vi "Front Panel.vi"(11 "GUI In":refnum<class "CRD Controls.lvclass">) -> ()   [LabVIEW 2015, in "CRD Controls.lvclass"]
uses:
  CRD Controls.lvclass
  Reusable/GUI/GUI.lvclass/GUI.ctl
  Reusable/Observer/Observer.lvclass/Observer.ctl
  CRDS/Data/cCRDS Data.lvclass
  Reusable/GUI/Accessors/Read RegEvent.vi
  Reusable/Observer/Read Data Queue.vi
  CRDS/Data/Read Humidifier T.vi
  CRDS/Data/Read Pressure.vi
  CRDS/Data/Read vData.vi
  CRDS/Data/Get Alicat Data.vi
  Reusable/Data/Data.lvclass
panel:
  in  "Med Humidity":T1
  in  "High Humidity":T1
  out "pidOut":cluster{"hum":sgl, "dry":sgl} caption="Humidifier PID \nOutput" {"dry" format="%#.2f"; "hum" format="%#.2f"}
  in  "orMFC":bool
  in  "lasEn":T2
  out "TRHin":cluster{"hum":sgl, "dry":sgl} caption="Humidifier \nTemperatures (degC)" {"dry" format="%#.2f"; "hum" format="%#.2f"}
  out "vaisalaData":T3 caption="Vaisala Data" {"ref 2"."TRH" format="%.2f"; "ref 2"."RH" format="%.2f"; "ref"."TRH" format="%.2f"; "ref"."RH" format="%.2f"; "dry"."TRH" format="%.2f"; "dry"."RH" format="%.2f"; "hum"."TRH" format="%.2g"; "hum"."RH" format="%.2g"}
  out "alctData":T4 caption="Alicat Data" {"purge"."P" format="%.2f"; "purge"."T" format="%.2f"; "purge"."Q" format="%.2f"; "hRH"."P" format="%.2f"; "hRH"."T" format="%.2f"; "hRH"."Q" format="%.2f"; "mRH"."P" format="%.2f"; "mRH"."T" format="%.2f"; "mRH"."Q" format="%.2f"; "dry"."P" format="%.2f"; "dry"."T" format="%.2f"; "dry"."Q" format="%.2f"; "denude"."P" format="%.2f"; "denude"."T" format="%.2f"; "denude"."Q" format="%.2f"}
  out "P":T5 caption="Pressure (mb)" {"ref 2" format="%#.2f"; "ref" format="%#.2f"; "dry" format="%#.2f"; "hum" format="%#.2f"}
  in  "Laser Controls":cluster{"f (Hz)":dbl, "Duty Cycle (%)":dbl}
  in  "crdFlows":T6 caption="Flow Rate Setpoints (LPM)" {"purge" max=5 format="%.2f"; "hRH" max=5 format="%.2f"; "mRH" max=5 format="%.2f"; "dry" max=5 format="%.2f"; "denude" max=5 format="%.2f"}
  # "CRD Controls"
  # "CRD Controller Data"
  # "Laser Enable"
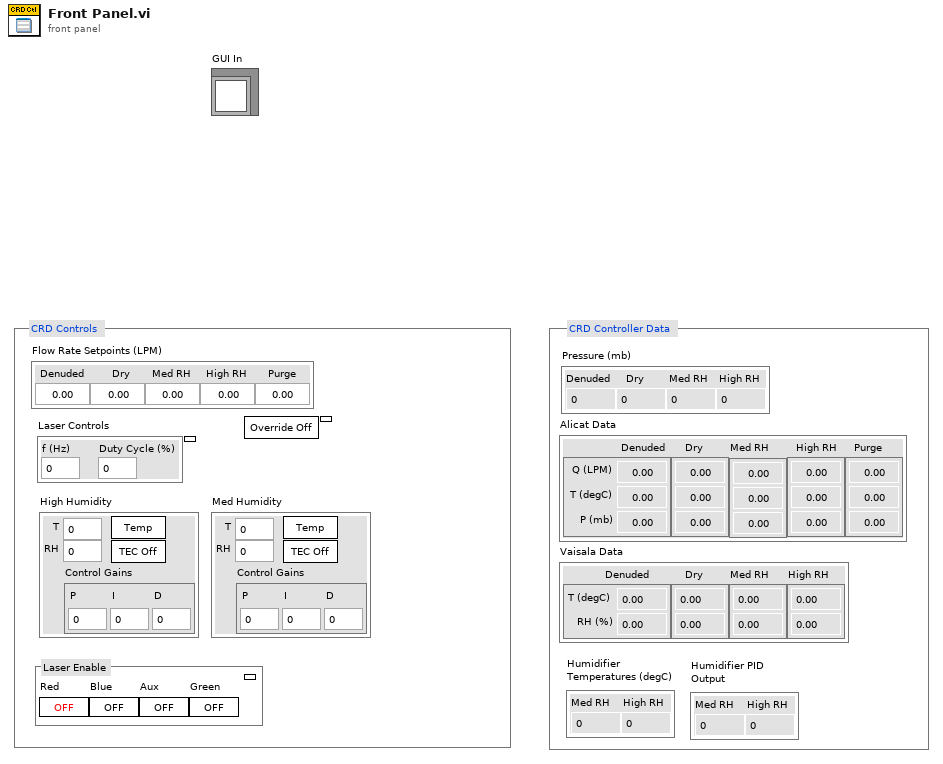
[diagram p1: front panel]
types:
  T1 = cluster{"T":dbl, "RH":dbl, "enable":bool, "ctl":bool, "Ctl Gains":cluster{"P":sgl, "I":sgl, "D":sgl}}
  T2 = cluster{"red":bool, "Blue":bool, "Aux":bool, "Green":bool}
  T3 = cluster{"hum":cluster{"RH":sgl, "TRH":sgl}, "dry":cluster{"RH":sgl, "TRH":sgl}, "ref":cluster{"RH":sgl, "TRH":sgl}, "ref 2":cluster{"RH":sgl, "TRH":sgl}}
  T4 = cluster{"denude":cluster{"Q":sgl, "T":sgl, "P":sgl}, "dry":cluster{"Q":sgl, "T":sgl, "P":sgl}, "mRH":cluster{"Q":sgl, "T":sgl, "P":sgl}, "hRH":cluster{"Q":sgl, "T":sgl, "P":sgl}, "purge":cluster{"Q":sgl, "T":sgl, "P":sgl}}
  T5 = cluster{"hum":sgl, "dry":sgl, "ref":sgl, "ref 2":sgl}
  T6 = cluster{"denude":sgl, "dry":sgl, "mRH":sgl, "hRH":sgl, "purge":sgl}
  T7 = enum8{"Enabled", "Disabled", "Disabled and Grayed Out"}
  T8 = cluster{"Array of Single[0]":sgl, "Array of Single[1]":sgl, "Array of Single[2]":sgl}
  T9 = cluster{"Numeric":sgl, "Numeric":sgl, "Numeric":sgl, "Numeric":sgl, "Numeric":sgl}
  T10 = cluster{"P":sgl, "T":sgl, "Q":sgl, "Q0":sgl, "Qsp":sgl}[]
  T11 = cluster{"Pressure[0]":sgl, "Pressure[1]":sgl, "Pressure[2]":sgl, "Pressure[3]":sgl}
  T12 = cluster{"vData[0]":cluster{"TRH":dbl, "RH":dbl}, "vData[1]":cluster{"TRH":dbl, "RH":dbl}, "vData[2]":cluster{"TRH":dbl, "RH":dbl}, "vData[3]":cluster{"TRH":dbl, "RH":dbl}}
  T13 = cluster{"P":sgl, "T":sgl, "Q":sgl, "Q0":sgl, "Qsp":sgl}
  T14 = cluster{"[0]":cluster{"Q":sgl, "T":sgl, "P":sgl}, "[1]":cluster{"Q":sgl, "T":sgl, "P":sgl}, "[2]":cluster{"Q":sgl, "T":sgl, "P":sgl}, "[3]":cluster{"Q":sgl, "T":sgl, "P":sgl}, "[4]":cluster{"Q":sgl, "T":sgl, "P":sgl}}
  T15 = cluster{"Array of Single[0]":sgl, "Array of Single[1]":sgl}
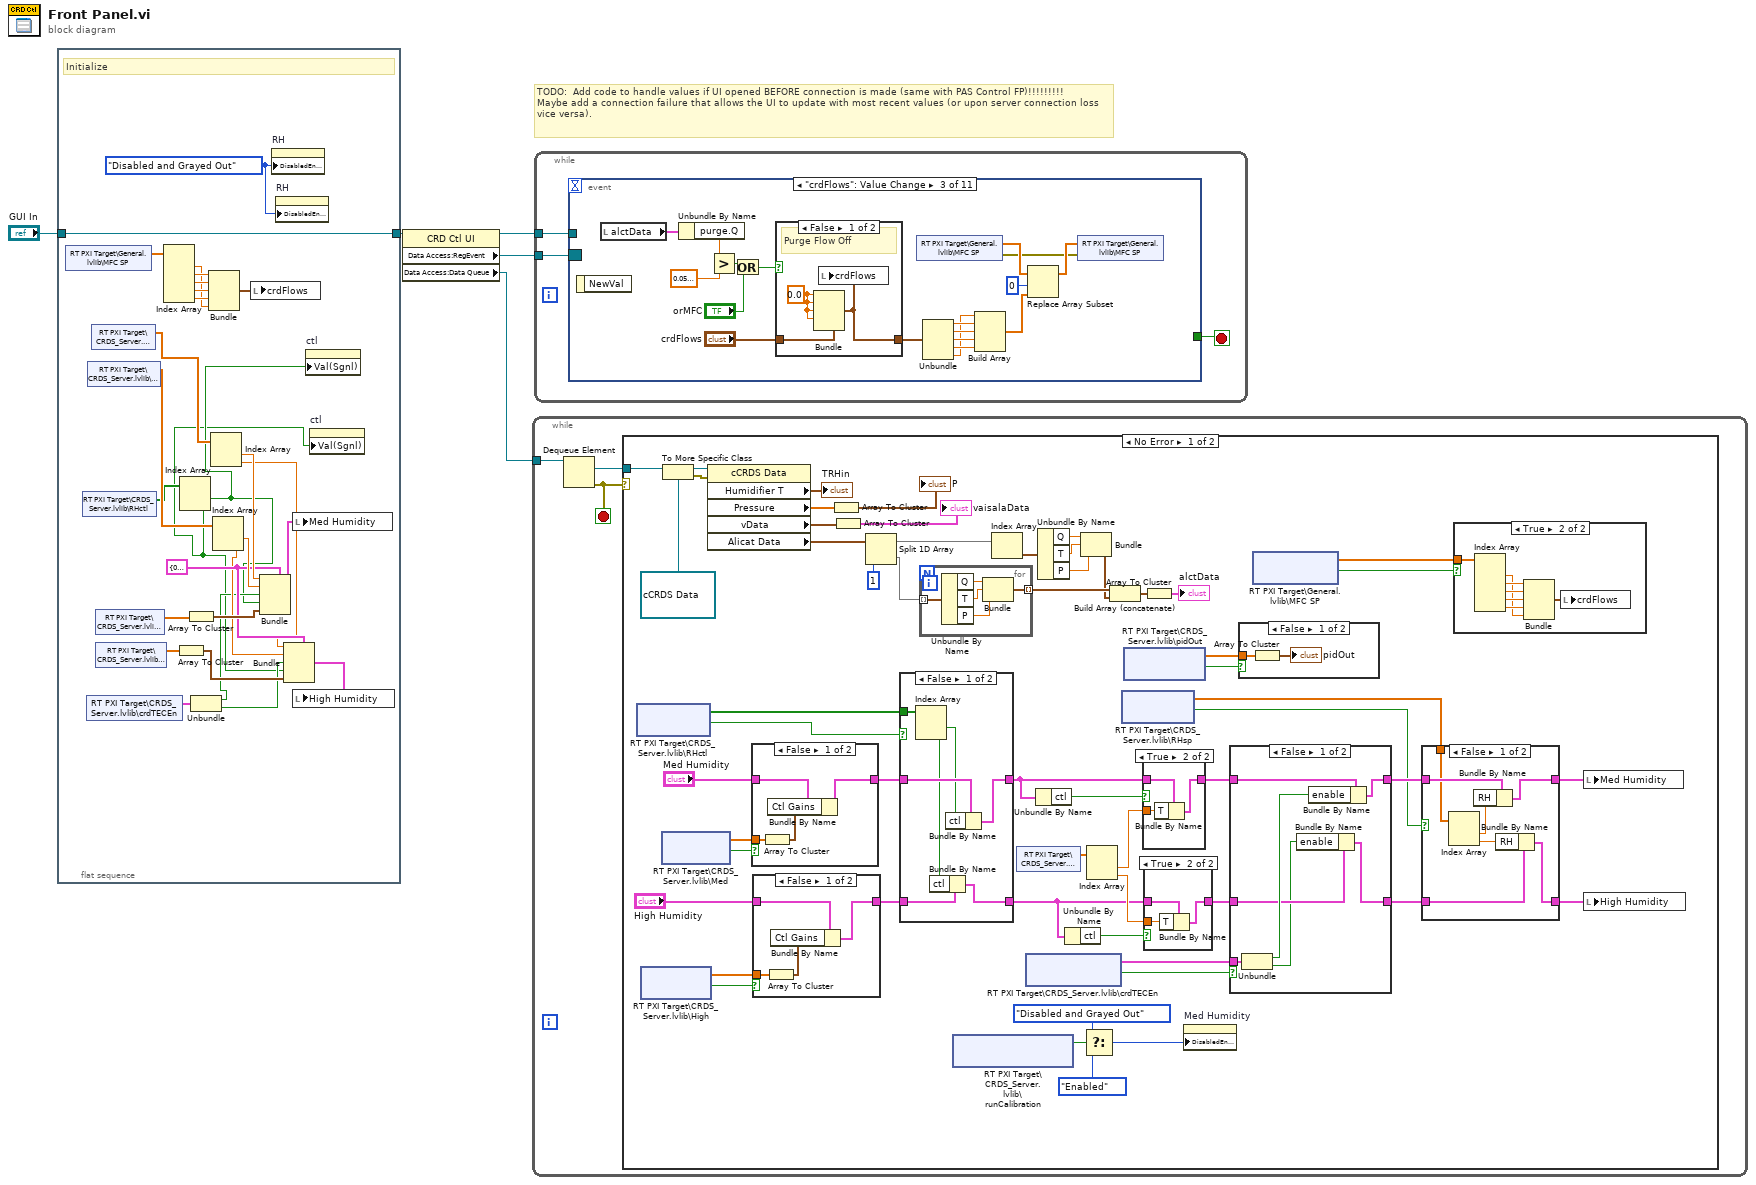
[diagram p0: block diagram]
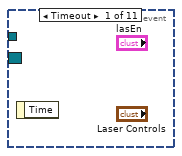
[diagram p2: hidden frame]
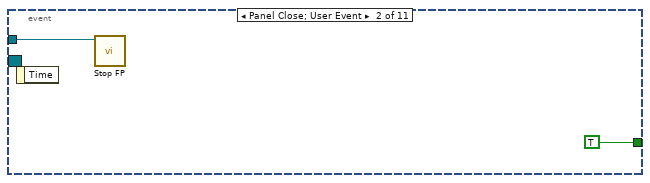
[diagram p3: hidden frame]
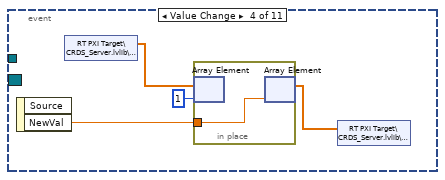
[diagram p5: hidden frame]
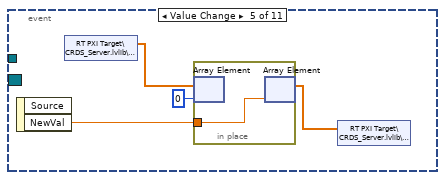
[diagram p6: hidden frame]
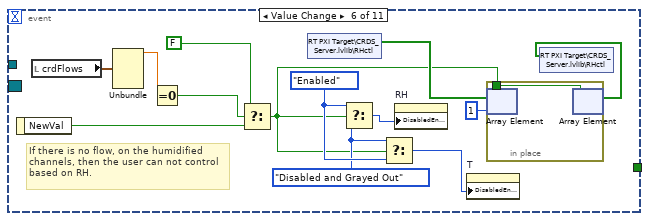
[diagram p7: hidden frame]
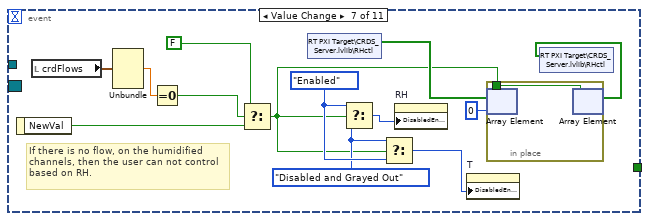
[diagram p8: hidden frame]
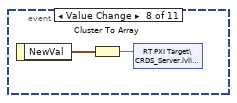
[diagram p9: hidden frame]
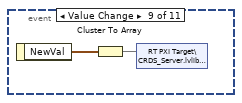
[diagram p10: hidden frame]
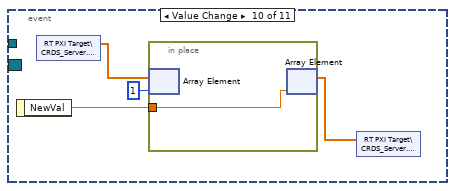
[diagram p11: hidden frame]
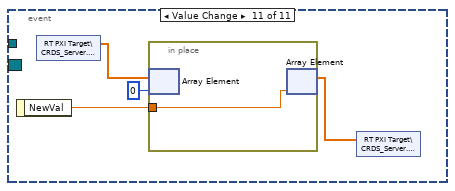
[diagram p12: hidden frame]
diagram:
  # "TODO:  Add code to handle values if UI opened BEFORE connection is made (same with PAS Control FP)!!!!!!!!!\nMaybe add a connection failure that allows the UI to update with most recent values (or upon server connection loss vice versa)."
  n1 = flat-sequence {
    tunnel: "GUI In" -> [w26]
    tunnel: [w26] -> w4
    frame #0 {
      w8 = T7."Disabled and Grayed Out" ("Disabled")
      w18 = T1 {"T"=0.0, "RH"=0.0, "enable"=FALSE, "ctl"=FALSE, "Ctl Gains"={"P"=3.0, "I"=10.0, "D"=0.1}} ("High Humidity")
      # "Initialize"
      n2 = shared-variable "RT PXI Target\\General.lvlib\\MFC SP"() -> (w33:sgl[])  [unwired: 1 in, 1 out]
      n3 = shared-variable "RT PXI Target\\CRDS_Server.lvlib\\RHctl"() -> (w14:bool[])  [unwired: 1 in, 1 out]
      n4 = shared-variable "RT PXI Target\\CRDS_Server.lvlib\\crdTECEn"() -> (w13:cluster{"med":bool, "high":bool})  [unwired: 1 in, 1 out]
      n5 = shared-variable "RT PXI Target\\CRDS_Server.lvlib\\RHsp"() -> (w22:sgl[])  [unwired: 1 in, 1 out]
      n6 = shared-variable "RT PXI Target\\CRDS_Server.lvlib\\Tsp"() -> (w23:sgl[])  [unwired: 1 in, 1 out]
      n7 = shared-variable "RT PXI Target\\CRDS_Server.lvlib\\Med"() -> (w25:sgl[])  [unwired: 1 in, 1 out]
      n8 = shared-variable "RT PXI Target\\CRDS_Server.lvlib\\High"() -> (w24:sgl[])  [unwired: 1 in, 1 out]
      n9 = Index Array(array=w33) -> (element #1=w28:sgl, element #2=w32:sgl, element #3=w31:sgl, element #4=w30:sgl, element #5=w29:sgl)  [unwired: 5 in]
      n10 = Array To Cluster(array=w24) -> (cluster=w17:T8)
      n11 = Index Array(array=w14) -> (element #1=w7:bool, element #2=w6:bool)  [unwired: 2 in]
      n12 = Array To Cluster(array=w25) -> (cluster=w21:T8)
      n13 = Unbundle(w13) -> ("med"=w12:bool, "high"=w11:bool)
      n14 = Bundle("Numeric"=w32, "Numeric"=w31, "Numeric"=w30, "Numeric"=w29, "Numeric"=w28) -> (w27:T9)  [unwired: 1 in]
      n15 = Index Array(array=w23) -> (element #1=w20:sgl, element #2=w16:sgl)  [unwired: 2 in]
      n16 = Index Array(array=w22) -> (element #1=w19:sgl, element #2=w15:sgl)  [unwired: 2 in]
      n17 = local write "crdFlows"(w27) -> ()
      n18 = Bundle(cluster=w18, "T"=w20, "RH"=w19, "enable"=w12, "ctl"=w7, "Ctl Gains"=w21) -> (w9:T1)
      n19 = property on="RH" class="DigNum (strict)"("DisabledEnum"=w8) -> ()  [unwired: 2 in, 2 out]
      n20 = property on="RH" class="DigNum (strict)"("DisabledEnum"=w8) -> ()  [unwired: 2 in, 2 out]
      n21 = Bundle(cluster=w18, "T"=w16, "RH"=w15, "enable"=w11, "ctl"=w6, "Ctl Gains"=w17) -> (w10:T1)
      n22 = local write "Med Humidity"(w9) -> ()
      n23 = local write "High Humidity"(w10) -> ()
      n24 = property on="ctl" class="Bool (strict)"("Val(Sgnl)"=w7) -> ()  [unwired: 2 in, 2 out]
      n25 = property on="ctl" class="Bool (strict)"("Val(Sgnl)"=w6) -> ()  [unwired: 2 in, 2 out]
    }
  }
  n26 = property class="CRD Ctl UI"(reference=w4) -> (reference out=w1:refnum<class "CRD Controls.lvclass">, "Data Access:RegEvent"=w3:refnum<event-registration>, "Data Access:Data Queue"=w2:refnum<queue>)  [unwired: 1 in, 1 out]
  n27 = while {
    tunnel: w2 -> [w36]
    stop <- w35 stop-if-true
    n28 = Dequeue Element(queue=w36) -> (element=w34:refnum<data-value>, error out=w35:errorcluster)  [unwired: 2 in, 2 out]
    n29 = case shown="No Error" w35 {
      tunnel: w34 -> [w75 _]
      frame No Error {
        n30 = shared-variable "RT PXI Target\\CRDS_Server.lvlib\\RHctl"() -> (w62:bool[], w64:bool)  [unwired: 2 in, 1 out]
        n31 = shared-variable "RT PXI Target\\CRDS_Server.lvlib\\High"() -> (w70:sgl[], w71:bool)  [unwired: 2 in, 1 out]
        n32 = shared-variable "RT PXI Target\\CRDS_Server.lvlib\\Med"() -> (w69:sgl[], w68:bool)  [unwired: 2 in, 1 out]
        n33 = To More Specific Class(target class=refnum<data-value> refnum ("element"), reference=w75) -> (specific class reference=w74:refnum<data-value>, error out=w73:errorcluster)  [unwired: 1 in]
        n34 = property class="cCRDS Data"(reference=w74, error in=w73) -> ("Humidifier T"=→"TRHin":cluster{"Hum 1":sgl, "Hum 2":sgl}, "Pressure"=w86:sgl[], "vData"=w85:cluster{"TRH":dbl, "RH":dbl}[], "Alicat Data"=w81:T10)  [unwired: 2 out]
        n35 = case shown="False" w68 {
          tunnel: w69 -> [w140 _]
          tunnel: "Med Humidity" -> [w139 w141]
          tunnel: [w137 w141] -> w60
          frame False {
            n36 = Array To Cluster(array=w140) -> (cluster=w138:T8)
            n37 = Bundle By Name(cluster=w139, "Ctl Gains"=w138) -> (w137:T1)
          }
          frame True {
          }
        }
        n38 = case shown="False" w71 {
          tunnel: w70 -> [w145 _]
          tunnel: "High Humidity" -> [w144 w146]
          tunnel: [w142 w146] -> w63
          frame False {
            n39 = Array To Cluster(array=w145) -> (cluster=w143:T8)
            n40 = Bundle By Name(cluster=w144, "Ctl Gains"=w143) -> (w142:T1)
          }
          frame True {
          }
        }
        n41 = Array To Cluster(array=w86) -> (cluster=→"P":T11)
        n42 = Array To Cluster(array=w85) -> (cluster=→"vaisalaData":T12)
        n43 = Split 1D Array(array=w81, index=1) -> (first subarray=w91:T10, second subarray=w92:T10)
        n44 = case shown="False" w64 {
          tunnel: w63 -> [w132 w134]
          tunnel: [w131 w134] -> w54
          tunnel: w62 -> [w129 _]
          tunnel: w60 -> [w130 w133]
          tunnel: [w126 w133] -> w53
          frame False {
            n45 = Index Array(array=w129) -> (element #1=w127:bool, element #2=w128:bool)  [unwired: 2 in]
            n46 = Bundle By Name(cluster=w132, "ctl"=w128) -> (w131:T1)
            n47 = Bundle By Name(cluster=w130, "ctl"=w127) -> (w126:T1)
          }
          frame True {
          }
        }
        n48 = for {
          tunnel: w92 -> [w151] mode=indexing
          tunnel: [w150] -> w90 mode=indexing
          n49 = Unbundle By Name(w151) -> ("Q"=w149:sgl, "T"=w148:sgl, "P"=w147:sgl)
          n50 = Bundle("Q"=w149, "T"=w148, "P"=w147) -> (w150:cluster{"Q":sgl, "T":sgl, "P":sgl})  [unwired: 1 in]
        }
        n51 = shared-variable "RT PXI Target\\CRDS_Server.lvlib\\runCalibration"() -> (w42:bool)  [unwired: 2 in, 2 out]
        n52 = Index Array(array=w91) -> (element=w87:T13)  [unwired: 1 in]
        n53 = shared-variable "RT PXI Target\\CRDS_Server.lvlib\\Tsp"() -> (w57:sgl[])  [unwired: 1 in, 1 out]
        n54 = shared-variable "RT PXI Target\\CRDS_Server.lvlib\\crdTECEn"() -> (w49:cluster{"med":bool, "high":bool}, w52:bool)  [unwired: 2 in, 1 out]
        n55 = Unbundle By Name(w53) -> ("ctl"=w59:bool)
        n56 = Unbundle By Name(w87) -> ("Q"=w84:sgl, "T"=w83:sgl, "P"=w82:sgl)
        n57 = Unbundle By Name(w54) -> ("ctl"=w58:bool)
        n58 = Bundle("Q"=w84, "T"=w83, "P"=w82) -> (w80:cluster{"Q":sgl, "T":sgl, "P":sgl})  [unwired: 1 in]
        n59 = Select(t=T7."Disabled and Grayed Out" ("Disabled"), s=w42, f=T7."Enabled" ("Disabled")) -> (s? t:f=w39:T7)
        n60 = Index Array(array=w57) -> (element #1=w56:sgl, element #2=w55:sgl)  [unwired: 2 in]
        n61 = Build Array (concatenate)(w90, w80) -> (w89:cluster{"Q":sgl, "T":sgl, "P":sgl}[])
        n62 = shared-variable "RT PXI Target\\CRDS_Server.lvlib\\RHsp"() -> (w45:sgl[], w46:bool)  [unwired: 2 in, 1 out]
        n63 = shared-variable "RT PXI Target\\CRDS_Server.lvlib\\pidOut"() -> (w67:sgl[], w66:bool)  [unwired: 2 in, 1 out]
        n64 = case shown="True" w59 {
          tunnel: w56 -> [_ w124]
          tunnel: w53 -> [w122 w125]
          tunnel: [w122 w123] -> w51
          frame False {
          }
          frame True {
            n65 = Bundle By Name(cluster=w125, "T"=w124) -> (w123:T1)
          }
        }
        n66 = Array To Cluster(array=w89) -> (cluster=→"alctData":T14)
        n67 = case shown="True" w58 {
          tunnel: w55 -> [_ w120]
          tunnel: w54 -> [w118 w121]
          tunnel: [w118 w119] -> w50
          frame False {
          }
          frame True {
            n68 = Bundle By Name(cluster=w121, "T"=w120) -> (w119:T1)
          }
        }
        n69 = property on="Med Humidity" class="Clust (strict)"("DisabledEnum"=w39) -> ()  [unwired: 2 in, 2 out]
        n70 = case shown="False" w52 {
          tunnel: w51 -> [w114 w117]
          tunnel: w50 -> [w111 w116]
          tunnel: [w113 w117] -> w48
          tunnel: [w109 w116] -> w47
          tunnel: w49 -> [w115 _]
          frame False {
            n71 = Unbundle(w115) -> ("med"=w112:bool, "high"=w110:bool)
            n72 = Bundle By Name(cluster=w111, "enable"=w110) -> (w109:T1)
            n73 = Bundle By Name(cluster=w114, "enable"=w112) -> (w113:T1)
          }
          frame True {
          }
        }
        n74 = case shown="False" w66 {
          tunnel: w67 -> [w136 _]
          frame False {
            n75 = Array To Cluster(array=w136) -> (cluster=→"pidOut":T15)
          }
          frame True {
          }
        }
        n76 = shared-variable "RT PXI Target\\General.lvlib\\MFC SP"() -> (w37:sgl[], w38:bool)  [unwired: 2 in, 1 out]
        n77 = case shown="False" w46 {
          tunnel: w48 -> [w106 w108]
          tunnel: [w105 w108] -> w43
          tunnel: [w104 w107] -> w44
          tunnel: w47 -> [w103 w107]
          tunnel: w45 -> [w102 _]
          frame False {
            n78 = Index Array(array=w102) -> (element #1=w101:sgl, element #2=w100:sgl)  [unwired: 2 in]
            n79 = Bundle By Name(cluster=w106, "RH"=w101) -> (w105:T1)
            n80 = Bundle By Name(cluster=w103, "RH"=w100) -> (w104:T1)
          }
          frame True {
          }
        }
        n81 = case shown="True" w38 {
          tunnel: w37 -> [_ w99]
          frame False {
          }
          frame True {
            n82 = Index Array(array=w99) -> (element #1=w94:sgl, element #2=w98:sgl, element #3=w97:sgl, element #4=w96:sgl, element #5=w95:sgl)  [unwired: 5 in]
            n83 = Bundle("Numeric"=w98, "Numeric"=w97, "Numeric"=w96, "Numeric"=w95, "Numeric"=w94) -> (w93:T9)  [unwired: 1 in]
            n84 = local write "crdFlows"(w93) -> ()
          }
        }
        n85 = local write "Med Humidity"(w43) -> ()
        n86 = local write "High Humidity"(w44) -> ()
      }
      frame Error {
      }
    }
  }
  n87 = while {
    tunnel: w3 -> [w153]
    tunnel: w1 -> [w152]
    stop <- w154 stop-if-true
    n88 = event shown="[2] \"crdFlows\": Value Change" {
      selector: w153 -> [_ _ _ _ _ _ _ _ _ _ _]
      dyn-events: _ -> [_ _ _ _ _ _ _ _ _ _ _]
      timeout: _ -> [_ _ _ _ _ _ _ _ _ _ _]
      tunnel: [_ TRUE _ _ _ _ _ _ _ _ _] -> w154
      tunnel: w152 -> [_ w155 _ _ _ _ _ _ _ _ _]
      event Timeout {
        n89 = event-data() -> ()  [unwired: 1 in, 1 out]
      }
      event Panel Close; User Event {
        n90 = event-data() -> ()  [unwired: 1 in, 1 out]
        n91 = call-dynamic "Stop FP.vi"("GUI in"=w155) -> ()  [unwired: 9 in, 2 out]
      }
      event "crdFlows": Value Change {
        n92 = event-data() -> ()  [unwired: 1 in, 1 out]
        n93 = local read "alctData"() -> (w161:T4)
        n94 = Unbundle By Name(w161) -> ("purge.Q"=w163:sgl)
        n95 = Greater?(x=w163, y=sgl 0.05) -> (0:w158:bool)
        n96 = Or(x=w158, y="orMFC") -> (x .or. y?=w157:bool)
        n97 = case shown="False" w157 {
          tunnel: "crdFlows" -> [w177 w178]
          tunnel: [w175 w178] -> w162
          frame False {
            w176 = sgl 0.0 ("denude")
            # "Purge Flow Off"
            n98 = Bundle(cluster=w177, "denude"=w176, "dry"=w176, "mRH"=w176, "hRH"=w176) -> (w175:T6)  [unwired: 1 in]
            n99 = local write "crdFlows"(w175) -> ()
          }
          frame True {
          }
        }
        n100 = shared-variable "RT PXI Target\\General.lvlib\\MFC SP"() -> (w171:sgl[], error out=w165:errorcluster)  [unwired: 1 in]
        n101 = Unbundle(w162) -> ("denude"=w167:sgl, "dry"=w168:sgl, "mRH"=w169:sgl, "hRH"=w170:sgl, "purge"=w166:sgl)
        n102 = Build Array(w166, w167, w168, w169, w170) -> (w173:sgl[])
        n103 = Replace Array Subset(array=w171, new element=w173, index=0) -> (w172:sgl[])
        n104 = shared-variable "RT PXI Target\\General.lvlib\\MFC SP"(w172, error in=w165) -> ()  [unwired: 1 out]
      }
      event "High Humidity.RH": Value Change {
        n105 = event-data() -> ("NewVal"=w179:dbl)  [unwired: 1 in, 1 out]
        n106 = shared-variable "RT PXI Target\\CRDS_Server.lvlib\\RHsp"() -> (w182:sgl[])  [unwired: 1 in, 1 out]
        n107 = in-place {
          in-place-border: w179 -> [w183]
          n108 = in-place-array #1(w182, 1) -> ()  [unwired: 1 out]
          n109 = in-place-array #1(w183) -> (w181:sgl[])  [unwired: 1 out]
        }
        n110 = shared-variable "RT PXI Target\\CRDS_Server.lvlib\\RHsp"(w181) -> ()  [unwired: 1 in, 1 out]
      }
      event "Med Humidity.RH": Value Change {
        n111 = event-data() -> ("NewVal"=w184:dbl)  [unwired: 1 in, 1 out]
        n112 = shared-variable "RT PXI Target\\CRDS_Server.lvlib\\RHsp"() -> (w187:sgl[])  [unwired: 1 in, 1 out]
        n113 = in-place {
          in-place-border: w184 -> [w188]
          n114 = in-place-array #2(w187, 0) -> ()  [unwired: 1 out]
          n115 = in-place-array #2(w188) -> (w186:sgl[])  [unwired: 1 out]
        }
        n116 = shared-variable "RT PXI Target\\CRDS_Server.lvlib\\RHsp"(w186) -> ()  [unwired: 1 in, 1 out]
      }
      event "High Humidity.ctl": Value Change {
        w199 = T7."Disabled and Grayed Out" ("Disabled")
        w200 = T7."Enabled" ("Disabled")
        # "If there is no flow, on the humidified channels, then the user can not control based on RH."
        n117 = event-data() -> ("NewVal"=w196:bool)  [unwired: 1 in]
        n118 = local read "crdFlows"() -> (w197:T6)
        n119 = Unbundle(w197) -> ("denude"=w189:sgl)  [unwired: 4 out]
        n120 = Equal To 0?(x=w189) -> (x = 0?=w198:bool)
        n121 = Select(t=FALSE, s=w198, f=w196) -> (s? t:f=w192:bool)
        n122 = shared-variable "RT PXI Target\\CRDS_Server.lvlib\\RHctl"() -> (w195:bool[])  [unwired: 1 in, 1 out]
        n123 = Select(t=w200, s=w192, f=w199) -> (s? t:f=w191:T7)
        n124 = Select(t=w199, s=w192, f=w200) -> (s? t:f=w190:T7)
        n125 = property on="RH" class="DigNum (strict)"("DisabledEnum"=w191) -> ()  [unwired: 2 in, 2 out]
        n126 = property on="T" class="DigNum (strict)"("DisabledEnum"=w190) -> ()  [unwired: 2 in, 2 out]
        n127 = in-place {
          in-place-border: w192 -> [w202]
          n128 = in-place-array #3(w195, 1) -> ()  [unwired: 1 out]
          n129 = in-place-array #3(w202) -> (w193:bool[])  [unwired: 1 out]
        }
        n130 = shared-variable "RT PXI Target\\CRDS_Server.lvlib\\RHctl"(w193) -> ()  [unwired: 1 in, 1 out]
      }
      event "Med Humidity.ctl": Value Change {
        w213 = T7."Disabled and Grayed Out" ("Disabled")
        w214 = T7."Enabled" ("Disabled")
        # "If there is no flow, on the humidified channels, then the user can not control based on RH."
        n131 = event-data() -> ("NewVal"=w210:bool)  [unwired: 1 in]
        n132 = local read "crdFlows"() -> (w211:T6)
        n133 = Unbundle(w211) -> ("mRH"=w203:sgl)  [unwired: 4 out]
        n134 = Equal To 0?(x=w203) -> (x = 0?=w212:bool)
        n135 = Select(t=FALSE, s=w212, f=w210) -> (s? t:f=w206:bool)
        n136 = shared-variable "RT PXI Target\\CRDS_Server.lvlib\\RHctl"() -> (w209:bool[])  [unwired: 1 in, 1 out]
        n137 = Select(t=w214, s=w206, f=w213) -> (s? t:f=w205:T7)
        n138 = Select(t=w213, s=w206, f=w214) -> (s? t:f=w204:T7)
        n139 = property on="RH" class="Digital (strict)"("DisabledEnum"=w205) -> ()  [unwired: 2 in, 2 out]
        n140 = property on="T" class="Digital (strict)"("DisabledEnum"=w204) -> ()  [unwired: 2 in, 2 out]
        n141 = in-place {
          in-place-border: w206 -> [w216]
          n142 = in-place-array #4(w209, 0) -> ()  [unwired: 1 out]
          n143 = in-place-array #4(w216) -> (w207:bool[])  [unwired: 1 out]
        }
        n144 = shared-variable "RT PXI Target\\CRDS_Server.lvlib\\RHctl"(w207) -> ()  [unwired: 1 in, 1 out]
      }
      event "Med Humidity.Ctl Gains": Value Change {
        n145 = event-data() -> ("NewVal"=w218:cluster{"P":sgl, "I":sgl, "D":sgl})  [unwired: 1 in]
        n146 = Cluster To Array(cluster=w218) -> (array=w217:sgl[])
        n147 = shared-variable "RT PXI Target\\CRDS_Server.lvlib\\Med"(w217) -> ()  [unwired: 1 in, 1 out]
      }
      event "High Humidity.Ctl Gains": Value Change {
        n148 = event-data() -> ("NewVal"=w219:cluster{"P":sgl, "I":sgl, "D":sgl})  [unwired: 1 in]
        n149 = Cluster To Array(cluster=w219) -> (array=w220:sgl[])
        n150 = shared-variable "RT PXI Target\\CRDS_Server.lvlib\\High"(w220) -> ()  [unwired: 1 in, 1 out]
      }
      event "High Humidity.T": Value Change {
        n151 = event-data() -> ("NewVal"=w222:dbl)  [unwired: 1 in]
        n152 = shared-variable "RT PXI Target\\CRDS_Server.lvlib\\Tsp"() -> (w224:sgl[])  [unwired: 1 in, 1 out]
        n153 = in-place {
          in-place-border: w222 -> [w225]
          n154 = in-place-array #5(w224, 1) -> ()  [unwired: 1 out]
          n155 = in-place-array #5(w225) -> (w221:sgl[])  [unwired: 1 out]
        }
        n156 = shared-variable "RT PXI Target\\CRDS_Server.lvlib\\Tsp"(w221) -> ()  [unwired: 1 in, 1 out]
      }
      event "Med Humidity.T": Value Change {
        n157 = event-data() -> ("NewVal"=w227:dbl)  [unwired: 1 in]
        n158 = shared-variable "RT PXI Target\\CRDS_Server.lvlib\\Tsp"() -> (w229:sgl[])  [unwired: 1 in, 1 out]
        n159 = in-place {
          in-place-border: w227 -> [w230]
          n160 = in-place-array #6(w229, 0) -> ()  [unwired: 1 out]
          n161 = in-place-array #6(w230) -> (w226:sgl[])  [unwired: 1 out]
        }
        n162 = shared-variable "RT PXI Target\\CRDS_Server.lvlib\\Tsp"(w226) -> ()  [unwired: 1 in, 1 out]
      }
    }
  }
